vi "Finish.vi"   [LabVIEW 2015]
doc: "This VI is called just before exiting. It is expected to close I/O refnum, save collected data, etc."
uses:
  <vilib>/Rock Robotics/WPI/Utilities/WPI_GetSetVariantRefNum.vi
types:
  T1 = typedef "WPI_JoystickDevRef.ctl" = cluster{"Device":T2}
  T2 = typedef "WPI_JoystickDeviceEnum.ctl" = enum16{"USB 0", "USB 1", "USB 2", "USB 3", "USB 4", "USB 5"}
  T3 = typedef "WPI_RobotDriveDevRef.ctl" = cluster{"DevStatus":errorcluster, "Motors[]":T4[], "Square Inputs":bool, "Max Output":dbl}
  T4 = typedef "WPI_MotorControlDeviceRef.ctl" = cluster{"DeviceStatus":errorcluster, "Type":T5, "PWM":cluster{"PWM Channel":T6, "DeadBand":T7}, "CAN":cluster{"Device Number":u8, "Control Mode":T8, "Semaphore":T9, "Max Vout":dbl, "TalonSRX Control Mode":T10}, "Invert":bool}
  T5 = typedef "WPI_MotorControlType.ctl" = enum16{"PWM", "CAN", "CANTalonSRX"}
  T6 = typedef "FPGA_DIOPWMChannel.ctl" = enum8{"PWM 0", "PWM 1", "PWM 2", "PWM 3", "PWM 4", "PWM 5", "PWM 6", "PWM 7", "PWM 8", "PWM 9", "PWM MXP 0", "PWM MXP 1", "PWM MXP 2", "PWM MXP 3", "PWM MXP 4", "PWM MXP 5", "PWM MXP 6", "PWM MXP 7", "PWM MXP 8", "PWM MXP 9", "Invalid"}
  T7 = typedef "WPI_PWMDeadband.ctl" = cluster{"Name":string, "maxPositivePwm":i32, "minPositivePwm":i32, "centerPwm":i32, "maxNegativePwm":i32, "minNegativePwm":i32, "angularRange":u16}
  T8 = typedef "WPI_CANJaguar_ControlMode.ctl" = enum8{"Percent VBus", "Current", "Speed", "Position", "Voltage"}
  T9 = typedef "Semaphore RefNum" = refnum<k1>
  T10 = typedef "WPI_CANTalonSRX_APIControlMode.ctl" = enum8{"Percent VBus", "Speed", "Position", "Slave", "Unchanged / Invalid", "Voltage Compensation", "Current", "Motion Profile"}
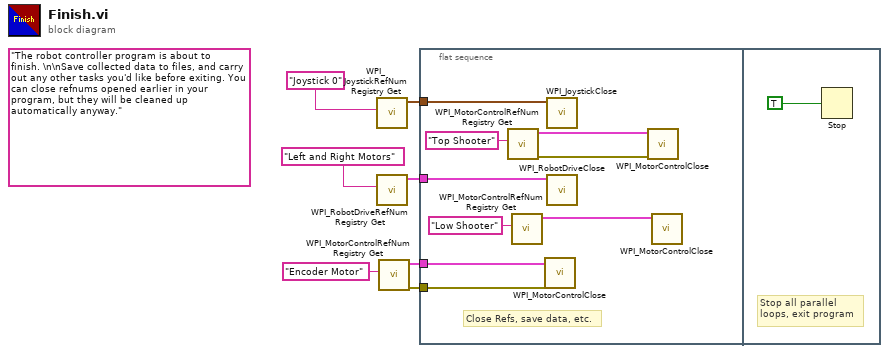
[diagram p0: block diagram]
diagram:
  (unwired) "The robot controller program is about to finish. \n\nSave collected data to files, and carry out any other tasks you'd like before exiting. You can close refnums opened earlier in your program, but they will be cleaned up automatically anyway."
  n1 = call <vilib>:"WPI_JoystickRefNum Registry Get.vi"("refnum name"="Joystick 0") -> ("JoystickDevRef"=w4:T1)  [unwired: 1 in, 9 out]
  n2 = call <vilib>:"WPI_RobotDriveRefNum Registry Get.vi"("refnum name"="Left and Right Motors") -> ("RobotDriveDevRef"=w5:T3)  [unwired: 1 in, 9 out]
  n3 = call <vilib>:"WPI_MotorControlRefNum Registry Get.vi"("refnum name"="Encoder Motor") -> ("error out"=w1:errorcluster, "MotorControlDevRef"=w2:T4)  [unwired: 9 in]
  n4 = flat-sequence {
    tunnel: w5 -> [w16]
    tunnel: w4 -> [w15]
    tunnel: w2 -> [w14]
    tunnel: w1 -> [w13]
    frame #0 {
      # "Close Refs, save data, etc."
      n5 = call <vilib>:"WPI_MotorControlRefNum Registry Get.vi"("refnum name"="Top Shooter") -> ("error out"=w12:errorcluster, "MotorControlDevRef"=w11:T4)  [unwired: 9 in]
      n6 = call <vilib>:"WPI_MotorControlRefNum Registry Get.vi"("refnum name"="Low Shooter") -> ("MotorControlDevRef"=w9:T4)  [unwired: 9 in, 1 out]
      n7 = call <vilib>:"WPI_MotorControlClose.vi"("error in (no error)"=w13, "MotorControlDevRef"=w14) -> ()  [unwired: 9 in, 1 out]
      n8 = call <vilib>:"WPI_JoystickClose.vi"("JoystickDevRef"=w15) -> ()  [unwired: 11 out]
      n9 = call <vilib>:"WPI_RobotDriveClose.vi"("RobotDriveDevRef"=w16) -> ()  [unwired: 1 in, 10 out]
      n10 = call <vilib>:"WPI_MotorControlClose.vi"("error in (no error)"=w12, "MotorControlDevRef"=w11) -> ()  [unwired: 9 in, 1 out]
      n11 = call <vilib>:"WPI_MotorControlClose.vi"("MotorControlDevRef"=w9) -> ()  [unwired: 10 in, 1 out]
    }
    frame #1 {
      # "Stop all parallel\nloops, exit program"
      n12 = Stop(stop? (T)=TRUE ("Quit")) -> ()
    }
  }
